vi "Read Section - Array (DBL).vi"(4 "Default":dbl[](array[numeric]), 6 "Create file if not found? (T)":bool=TRUE, 8 "error in (no error)":errorcluster, 9 "key":string, 10 "section":string, 11 "Path":path) -> (0 "error out":errorcluster, 3 "value":dbl[](array[numeric]))   [LabVIEW 2019, in "TSC File IO.lvlib"]
doc: "This VI will read a section/key configuration file and return:\n<b>array of doubles</b>\n\nInputs:\n-Path [path] - a path to the file\n-section [string] - the section string in the configuration file\n-key [string] - the key to be read in the configuration file\n-error in\n\nOutputs:\n-value [array of DBL] - the output data read\n-error out\n\n<b>Code Developed By:</b>\nDaniel Coons\nTechnology Service Corporation\n1983 S Liberty Drive\nBloomington, IN 47403\nwww.tsc.com\\atcs"
uses:
  TSC File IO.lvlib
  <vilib>/Utility/config.llb/Read Key (String).vi
  <vilib>/Utility/config.llb/NI_LVConfig.lvlib
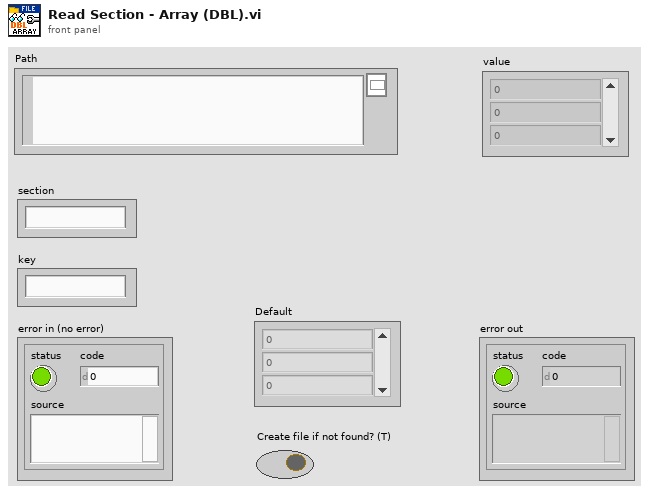
[diagram p1: front panel]
types:
  T1 = typedef "NI_LVConfig.lvlib/Config Data RefNum.ctl" = refnum<k1>
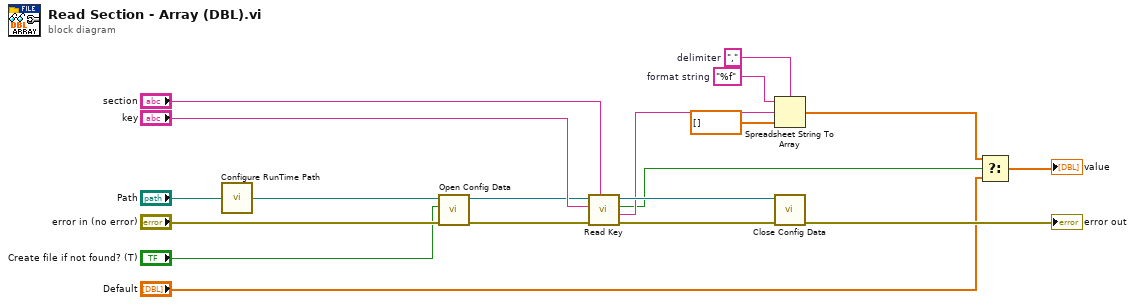
[diagram p0: block diagram]
diagram:
  w9 = "%f"  # format string
  w10 = ","  # delimiter
  n1 = call "Configure RunTime Path.vi"("Input Path"="Path") -> ("Updated Path"=w6:path)
  n2 = call <vilib>:"Open Config Data.vi"("error in (no error)"="error in (no error)", "create file if necessary (T)"="Create file if not found? (T)", "configuration file path"=w6) -> ("error out"=w12:errorcluster, "refnum"=w13:T1)  [unwired: 6 in, 1 out]
  n3 = call-poly <vilib>:"Read Key.vi"("section"="section", "error in (no error)"=w12, "key"="key", "refnum"=w13) -> ("error out"=w7:errorcluster, "value"=w11:string, "found?"=w4:bool, "refnum out"=w14:T1)  [unwired: 4 in]
  n4 = Spreadsheet String To Array(delimiter (Tab)=w10, format string=w9, spreadsheet string=w11, array type (2D Dbl)=dbl[] []) -> (array=w3:dbl[])
  n5 = call <vilib>:"Close Config Data.vi"("error in (no error)"=w7, "refnum"=w14) -> ("error out"=→"error out":errorcluster)  [unwired: 8 in, 1 out]
  n6 = Select(t=w3, s=w4, f="Default") -> (s? t:f=→"value":dbl[])
